vi "Is Clear.vi"(10 "Primary Direction":T1, 11 "View":i32[](array[numeric])) -> (2 "Clear Array Out":T1[](array[typedef]), 3 "Primary Clear Out":bool, 5 "Found Out":bool)   [LabVIEW 2017, in "AntFarm_MB.lvclass"]
uses:
  AntFarm_MB.lvclass
  Type Defs/Direction Enum.ctl
  Type Defs/SB Type Defs.lvlib
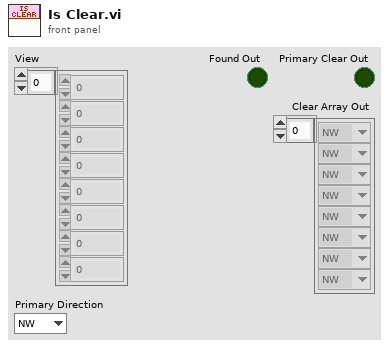
[diagram p1: front panel]
types:
  T1 = typedef "SB Type Defs.lvlib/Direction Enum.ctl" = enum16{"NW", "N", "NE", "E", "SE", "S", "SW", "W"}
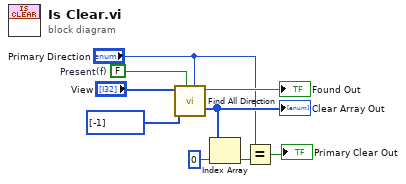
[diagram p0: block diagram]
diagram:
  w7 = FALSE  # Present(f)
  n1 = call "Find All Direction.vi"("Primary Direction"="Primary Direction", "Present(f) Not Present(t)"=w7, "Target Array"=i32[] [-1], "View"="View") -> ("Direction Array Out"=w5:T1[], "Found"=→"Found Out":bool)  [unwired: 6 in]
  "Clear Array Out" <- w5
  n2 = Index Array(array=w5, index=0) -> (element=w3:T1)
  n3 = Equal?(x="Primary Direction", y=w3) -> (x = y?=→"Primary Clear Out":bool)
